vi "Host_HealthCheck_Initializer.vi"(11 "Table in":refnum<vi>) -> ()   [LabVIEW 2017]
uses:
  Master/DAQ/Master_DataControl.ctl
  Master/DAQ/TypeDef_cRIOData.ctl
  Master/IMU/TypeDef_IMUData.ctl
  Master/CAN/TypeDef_BMSData.ctl
  Master/CAN/TypeDef_BMS_Status.ctl
  <vilib>/Utility/miscctls.llb/LVRowAndColumnTypeDef.ctl
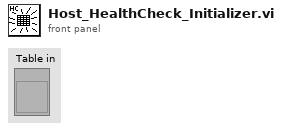
[diagram p1: front panel]
types:
  T1 = typedef "Master_DataControl.ctl" = cluster{"cRIO Data":T2, "IMU Data":T3, "BMS Data":T4, "Motor Data":cluster{"Motor":dbl}}
  T2 = typedef "TypeDef_cRIOData.ctl" = cluster{"Time (ms)":dbl, "24V Battery (V)":dbl, "LowV Current (I)":dbl, "Fiducial Sensor (V)":dbl, "PV Pressure (psig)":dbl, "Flow Sensor (V)":dbl, "Temp Fairing (F)":dbl, "Temp Reservoir (F)":dbl, "HallEffect Right (V)":dbl, "HallEffect Left (V)":dbl, "PT Tank (psig)":dbl, "PT Clamp Right (psig)":dbl, "PT Clamp Left (psig)":dbl, "PT Brake (psig)":dbl, "PT Cooling (psig)":dbl, "Displacement (ft)":dbl, "Velocity (ft/s)":dbl}
  T3 = typedef "TypeDef_IMUData.ctl" = cluster{"x acceleration (g)":dbl, "Pressure (psia)":dbl, "Temperature (F)":dbl}
  T4 = typedef "TypeDef_BMSData.ctl" = cluster{"Max Cell Voltage (V)":dbl, "Max Cell ID":dbl, "Min Cell Voltage (V)":dbl, "Min Cell ID":dbl, "State of Charge (%)":dbl, "Average Voltage (V)":dbl, "Voltage Delta (V)":dbl, "Pack Current (I)":dbl, "Pack Voltage (V)":dbl, "Max Resistance (Ohm)":dbl, "Min Resistance (Ohm)":dbl, "Average Resistance (Ohm)":dbl, "Delta Resistance (Ohm)":dbl, "BmsStatus":T5, "Highest Temperature(C)":dbl}
  T5 = typedef "TypeDef_BMS_Status.ctl" = cluster{"isFault":bool, "isolationMonitoring":bool}
  T6 = typedef "LVRowAndColumnTypeDef.ctl" = cluster{"Row":i32, "Column":i32}
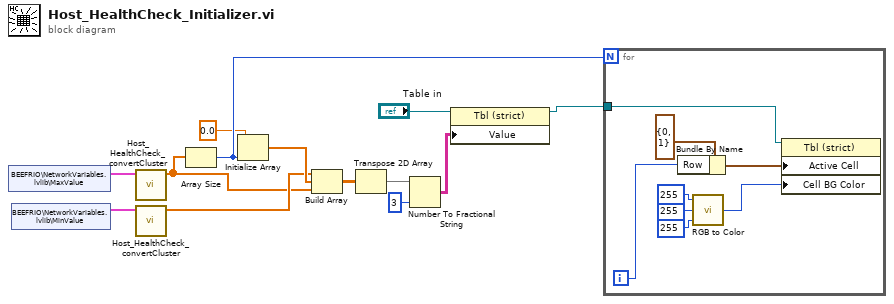
[diagram p0: block diagram]
diagram:
  n1 = shared-variable "BEEFRIO\\NetworkVariables.lvlib\\MaxValue"() -> (w8:T1)  [unwired: 1 in, 1 out]
  n2 = shared-variable "BEEFRIO\\NetworkVariables.lvlib\\MinValue"() -> (w7:T1)  [unwired: 1 in, 1 out]
  n3 = call "Host_HealthCheck_convertCluster.vi"("Data"=w8) -> ("Array"=w1:dbl[])  [unwired: 10 in]
  n4 = call "Host_HealthCheck_convertCluster.vi"("Data"=w7) -> ("Array"=w2:dbl[])  [unwired: 10 in]
  n5 = Array Size(array=w1) -> (size(s)=w13:i32)
  n6 = Initialize Array(0.0 ("element"), w13) -> (w10:dbl[])
  n7 = Build Array(w2, w10, w1) -> (w5:dbl[][])
  n8 = Transpose 2D Array(2D array=w5) -> (transposed array=w4:dbl[][])
  n9 = Number To Fractional String(number=w4, precision (6)=i16 3) -> (F-format string=w11:string[][])  [unwired: 2 in]
  n10 = property class="Tbl (strict)"(reference="Table in", "Value"=w11) -> (reference out=w12:refnum<vi>)  [unwired: 1 in, 1 out]
  n11 = for {
    N: w13 -> [_]
    tunnel: w12 -> [w15]
    i -> [w14]
    n12 = Bundle By Name(cluster=T6 {"Row"=0, "Column"=1} ("Active Cell:Active Cell"), "Row"=w14) -> (w17:T6)
    n13 = call <vilib>:"RGB to Color.vi"("B"=u8 255, "G"=u8 255, "R"=u8 255) -> ("Color"=w16:u32)
    n14 = property on="Property Node" class="Tbl (strict)"(reference=w15, "Active Cell"=w17, "Cell BG Color"=w16) -> ()  [unwired: 1 in, 2 out]
  }
